vi "PH_AxisGUI_BaseClass.PC Set Position in Units.vi"(0 "VI in":refnum<vi>, 2 "Axis":i32=-1, 3 "Position to set [Units]":dbl, 5 "error in (no error)":errorcluster) -> (14 "VI out":refnum<vi>, 19 "error out":errorcluster)   [LabVIEW 2014, in "PH_AxisGUI_BaseClass.lvlib"]
doc: "This VI acts on an axis."
uses:
  PH_AxisGUI_BaseClass.lvlib
  PH_Stepmotor_BaseClass/PH_Stepmotor_BaseClass.lvlib
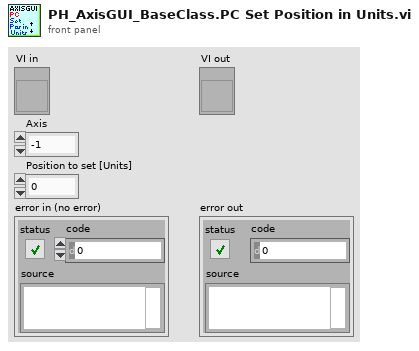
[diagram p1: front panel]
types:
  T1 = typedef "PH_Stepmotor_BaseClass.lvlib/PH_Stepmotor_BaseClass.Axis Address.ctl" = cluster{"Instance":string, "Motor Nr":i32}
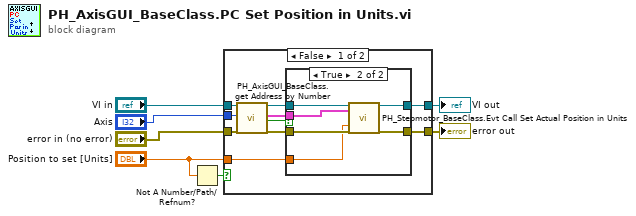
[diagram p0: block diagram]
diagram:
  n1 = Not A Number/Path/Refnum?(number/path/refnum="Position to set [Units]") -> (NaN/Path/Refnum?=w1:bool)
  n2 = case shown="False" w1 {
    tunnel: "VI in" -> [w16 w27]
    tunnel: [w14 w26] -> w6
    tunnel: [w13 w27] -> w5
    tunnel: "error in (no error)" -> [w12 w26]
    tunnel: "Axis" -> [w9 _]
    tunnel: "Position to set [Units]" -> [w8 _]
    frame False {
      n3 = call "PH_AxisGUI_BaseClass.get Address by Number.vi"("VI in"=w16, "Axis"=w9, "error in (no error)"=w12) -> ("VI out"=w17:refnum<vi>, "Address"=w11:T1, "Axis exists and is not moving?"=w10:bool, "error out"=w15:errorcluster)  [unwired: 12 in, 1 out]
      n4 = case shown="True" w10 {
        tunnel: [w19 w21] -> w13
        tunnel: [w18 w22] -> w14
        tunnel: w15 -> [w18 w25]
        tunnel: w17 -> [w19 w24]
        tunnel: w11 -> [_ w23]
        tunnel: w8 -> [_ w20]
        frame False {
        }
        frame True {
          n5 = call "PH_Stepmotor_BaseClass.Evt Call Set Actual Position in Units.vi"("i ref in"=w24, "Address"=w23, "Position to set [Units]"=w20, "error in"=w25) -> ("i ref out"=w21:refnum<vi>, "error out"=w22:errorcluster)  [unwired: 14 in]
        }
      }
    }
    frame True {
    }
  }
  "error out" <- w6
  "VI out" <- w5
